vi "mod_Modulo Integrator (real).vi"(6 "reset?":bool, 8 "initial y":dbl format="%.2f", 9 "modulo":dbl=-1.0 format="%.2f", 11 "x":dbl format="%.2f") -> (3 "y":dbl format="%.2f")   [LabVIEW 2020, in "niAMT.lvlib"]
uses:
  <vilib>/addons/Modulation/niAMT.lvlib
panel:
  # "H(z) = z/(z-1)"
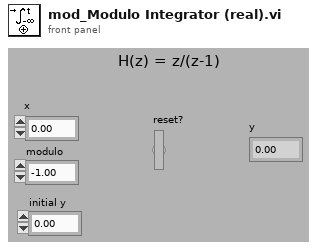
[diagram p1: front panel]
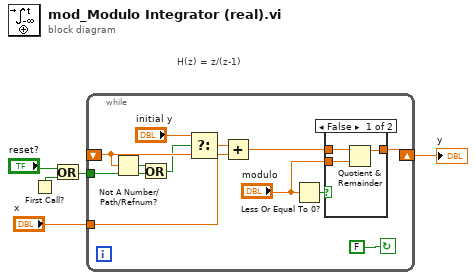
[diagram p0: block diagram]
diagram:
  # "H(z) = z/(z-1)"
  n1 = First Call?() -> (First Call?: T/F=w4:bool)
  n2 = Or(x="reset?", y=w4) -> (x .or. y?=w5:bool)
  n3 = while {
    tunnel: "x" -> [w12]
    tunnel: w5 -> [w6]
    shift-left: _ -> [w9]
    shift-right: [w11] -> w1
    stop <- FALSE continue-if-true
    n4 = Not A Number/Path/Refnum?(number/path/refnum=w9) -> (NaN/Path/Refnum?=w7:bool)
    n5 = Or(x=w7, y=w6) -> (x .or. y?=w8:bool)
    n6 = Select(t="initial y", s=w8, f=w9) -> (s? t:f=w13:dbl)
    n7 = Add(x=w13, y=w12) -> (x+y=w10:dbl)
    n8 = Less Or Equal To 0?(x="modulo") -> (x <= 0?=w16:bool)
    n9 = case shown="False" w16 {
      tunnel: [w19 w21] -> w11
      tunnel: w10 -> [w20 w21]
      tunnel: "modulo" -> [w18 _]
      frame False {
        n10 = Quotient & Remainder(x=w20, y=w18) -> (x-y*floor(x/y)=w19:dbl)  [unwired: 1 out]
      }
      frame True {
      }
    }
  }
  "y" <- w1
